vi "Get Minimal Maximal Size.vi"(7 "Vertical? [F, hor.]":bool, 8 "error in (no error)":errorcluster, 11 "Divider in":refnum<class "Divider.lvclass">) -> (0 "error out":errorcluster, 1 "Minimal size":i16, 2 "Maximal size":i16, 3 "IObject out":refnum<class "Divider.lvclass">)   [LabVIEW 2013, in "Divider.lvclass"]
doc: "Copyright 2018, Wiebe Walstra, wiebe@carya.nl."
uses:
  Divider.lvclass
  Divider.lvclass/Divider.ctl
  IObject.lvclass
  IContainer.lvclass
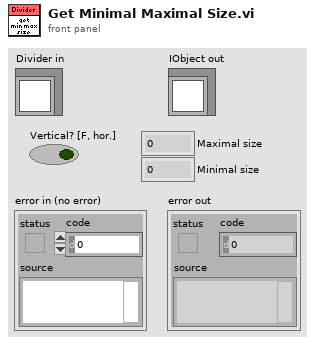
[diagram p1: front panel]
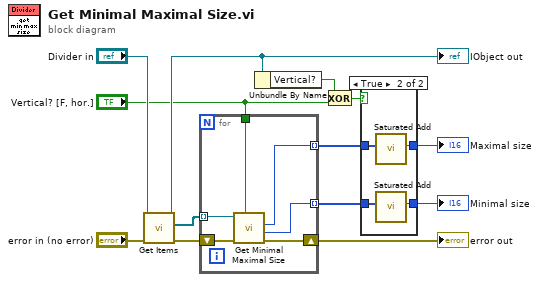
[diagram p0: block diagram]
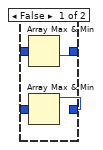
[diagram p2: hidden frame]
diagram:
  n1 = call "Get Items.vi"("error in (no error)"="error in (no error)", "IContainer in"="Divider in") -> ("error out"=w12:errorcluster, "Items"=w10:refnum<class "IObject.lvclass">[], "IContainer out"=w4:refnum<class "Divider.lvclass">)  [unwired: 7 in]
  "IObject out" <- w4
  n2 = for {
    tunnel: w10 -> [w19] mode=indexing
    shift-right: [w16] -> w11
    shift-left: w12 -> [w18]
    tunnel: [w17] -> w8 mode=indexing
    tunnel: [w14] -> w7 mode=indexing
    tunnel: "Vertical? [F, hor.]" -> [w15]
    n3 = call-dynamic "Get Minimal Maximal Size.vi"("Vertical? [F, hor.]"=w15, "error in (no error)"=w18, "IObject in"=w19) -> ("error out"=w16:errorcluster, "Minimal size"=w14:i16, "Maximal size"=w17:i16)  [unwired: 5 in, 1 out]
  }
  "error out" <- w11
  n4 = Unbundle By Name(w4) -> ("Vertical?"=w3:bool)
  n5 = Exclusive Or(1:"Vertical? [F, hor.]", 2:w3) -> (0:w1:bool)
  n6 = case shown="True" w1 {
    tunnel: w8 -> [w23 w27]
    tunnel: w7 -> [w21 w26]
    tunnel: [w20 w25] -> w6
    tunnel: [w22 w24] -> w5
    frame False {
      n7 = Array Max & Min(array=w23) -> (min value=w22:i16)  [unwired: 3 out]
      n8 = Array Max & Min(array=w21) -> (max value=w20:i16)  [unwired: 3 out]
    }
    frame True {
      n9 = call "Saturated Add.vi"("Sizes"=w27) -> ("Sum"=w24:i16)  [unwired: 10 in]
      n10 = call "Saturated Add.vi"("Sizes"=w26) -> ("Sum"=w25:i16)  [unwired: 10 in]
    }
  }
  "Maximal size" <- w5
  "Minimal size" <- w6
